vi "Test TCC Set Temperature Setpoint Triggers Setpoint Broadcast.vi"(8 "error in (no error)":errorcluster, 11 "Thermal Chamber Controller Test In":refnum<class "Thermal Chamber Controller Test.lvclass">) -> (0 "error out":errorcluster, 3 "Thermal Chamber Controller Test Out":refnum<class "Thermal Chamber Controller Test.lvclass">)   [LabVIEW 2020, in "Thermal Chamber Controller Test.lvclass"]
uses:
  Thermal Chamber Controller Test.lvclass
  C:/Program Files (x86)/National Instruments/LabVIEW 2020/vi.lib/Astemes/LUnit/Test Case.lvclass
  Thermal Chamber Controller/Thermal Chamber Controller.lvclass
  C:/Program Files (x86)/National Instruments/LabVIEW 2020/vi.lib/Astemes/Triarc Framework/Process/Process.lvclass
  <vilib>/Astemes/Triarc Framework/Process/Process.lvclass/Process.ctl
  <vilib>/Astemes/LUnit/Test Case.lvclass/Test Case.ctl
  <vilib>/Astemes/Triarc Framework/Broadcast Event Helpers/Execution timer.vi
  <vilib>/Astemes/Triarc Framework/Process/Private/SubVIs/Wait for finish.vi
  <vilib>/Astemes/Triarc Framework/Process/Private/SubVIs/Set Lifecycle State.vi
  <vilib>/Astemes/Triarc Framework/Process/Protected/Messaging/Send Message.vi
  <vilib>/Astemes/LUnit/Core/LUnit Test Case/Private/Append Pass Result.vi
  <vilib>/Astemes/LUnit/Core/LUnit Test Case/Private/Append Fail Result.vi
  <vilib>/Astemes/Triarc Framework/Process/Private/SubVIs/Handle Debug Data.vi
  <vilib>/Astemes/LUnit/Core/LUnit Test Case/Private/Run In UI.vi
  <vilib>/Utility/error.llb/Clear Errors.vi
  <vilib>/Astemes/Triarc Framework/Support/Dequeue Broadcast Message.vi
  <vilib>/Astemes/Triarc Framework/Process/Public/Lifecycle/Get Lifecycle State.vi
  <vilib>/Utility/error.llb/Error Cluster From Error Code.vi
  <vilib>/Astemes/Triarc Framework/Callback/Callback.lvclass
  <vilib>/Astemes/Triarc Framework/Process/Process.lvclass
  <vilib>/Astemes/LUnit/Test Case.lvclass
  <vilib>/Astemes/Triarc Framework/Broadcast Event Helpers/Broadcast Event Helpers.lvlib
panel:
  out "Message Data":variant
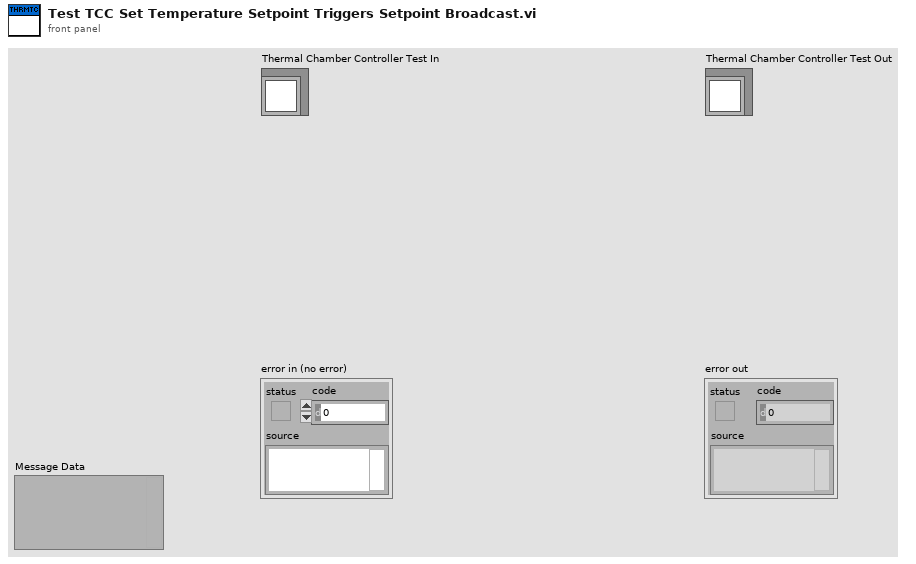
[diagram p1: front panel]
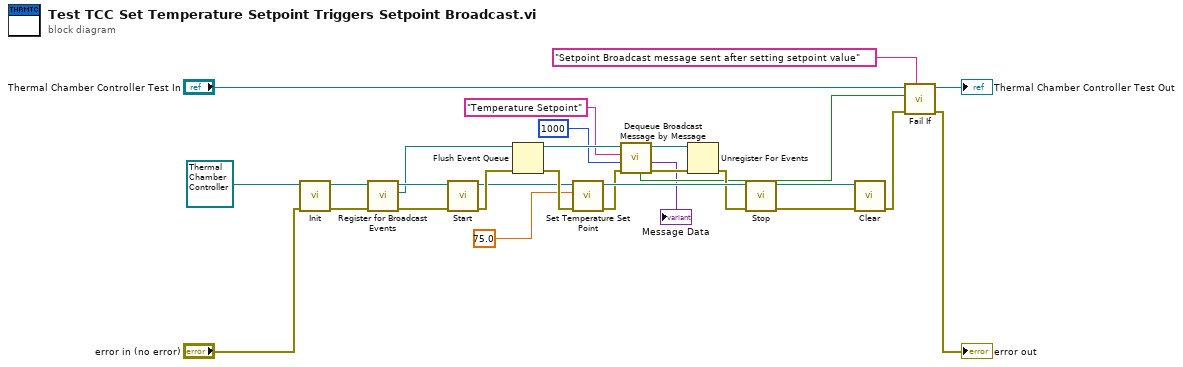
[diagram p0: block diagram]
diagram:
  n1 = call-dynamic "Init.vi"("error in (no error)"="error in (no error)", "View In"=refnum<class "Thermal Chamber Controller.lvclass"> refnum ("Thermal Chamber Controller.lvclass")) -> ("error out"=w21:errorcluster, "View Out"=w23:refnum<class "Thermal Chamber Controller.lvclass">)  [unwired: 8 in]
  n2 = call <vilib>:"Register for Broadcast Events.vi"("error in (no error)"=w21, "Process In"=w23) -> ("error out"=w20:errorcluster, "Event Registration Refnum Out"=w15:refnum<event-registration>, "Process Out"=w22:refnum<class "Thermal Chamber Controller.lvclass">)  [unwired: 7 in]
  n3 = call <vilib>:"Start.vi"("error in (no error)"=w20, "Process In"=w22) -> ("error out"=w27:errorcluster, "Process Out"=w5:refnum<class "Thermal Chamber Controller.lvclass">)  [unwired: 7 in, 1 out]
  n4 = Flush Event Queue(0:w15, 3:w27) -> (8:w14:refnum<event-registration>, 11:w16:errorcluster)  [unwired: 4 in, 1 out]
  n5 = call "Set Temperature Set Point.vi"("error in (no error)"=w16, "Temperature Set Point"=75.0, "Thermal Chamber Controller In"=w5) -> ("error out"=w18:errorcluster, "Thermal Chamber Controller Out"=w26:refnum<class "Thermal Chamber Controller.lvclass">)  [unwired: 7 in]
  n6 = call <vilib>:"Dequeue Broadcast Message by Message.vi"("error in (no error)"=w18, "Timeout (-1)"=1000, "Message"="Temperature Setpoint", "Event Registration Refnum"=w14) -> ("error out"=w17:errorcluster, "Message Data"=→"Message Data":variant, "Event Registration Refnum Out"=w12:refnum<event-registration>, "Timed Out?"=w10:bool)  [unwired: 3 in, 1 out]
  n7 = Unregister For Events(event registration refnum=w12, error in=w17) -> (error out=w13:errorcluster)
  n8 = call <vilib>:"Stop.vi"("error in (no error)"=w13, "Process In"=w26) -> ("error out"=w24:errorcluster, "Process Out"=w25:refnum<class "Thermal Chamber Controller.lvclass">)  [unwired: 7 in, 1 out]
  n9 = call-dynamic "Clear.vi"("error in (no error)"=w24, "View In"=w25) -> ("error out"=w19:errorcluster)  [unwired: 9 in]
  n10 = call <vilib>:"Fail If.vi"("Description"="Setpoint Broadcast message sent after setting setpoint value", "error in (no error)"=w19, "Fail?"=w10, "LUnit Test Case In"="Thermal Chamber Controller Test In") -> ("error out"=→"error out":errorcluster, "LUnit Test Case Out"=→"Thermal Chamber Controller Test Out":refnum<class "Thermal Chamber Controller Test.lvclass">)  [unwired: 6 in]
